vi "arduinoClose.vi"(1 "error in (no error)":errorcluster, 2 "VISA resource name out":refnum<visa-resource-name>) -> (0 "error out":errorcluster)   [LabVIEW 2021]
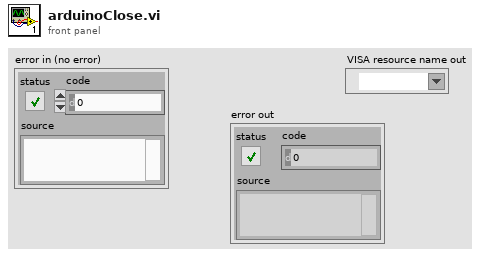
[diagram p1: front panel]
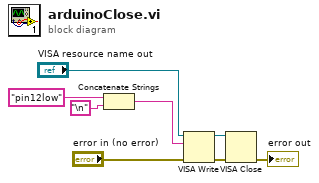
[diagram p0: block diagram]
diagram:
  n1 = Concatenate Strings("pin12low", "\n") -> (w6:string)
  n2 = VISA Write(VISA resource name="VISA resource name out", write buffer=w6, error in (no error)="error in (no error)") -> (VISA resource name out=w2:refnum<visa-resource-name>, error out=w3:errorcluster)  [unwired: 1 out]
  n3 = VISA Close(VISA resource name=w2, error in (no error)=w3) -> (error out=→"error out":errorcluster)
